vi "Tab Control(Calculator).vi"() -> ()   [LabVIEW 2012]
panel:
  in  "stop":bool
  in  "Tab Control":enum32{"ADD", "SUB", "MUL", "DIV"}(tab)
  out "Result":dbl
  in  "No2":dbl
  in  "NO1":dbl
  in  "NO1 2":dbl
  in  "No2 2":dbl
  out "Result 2":dbl
  in  "NO1 3":dbl
  in  "No2 3":dbl
  out "Result 3":dbl
  in  "NO1 4":dbl
  in  "No2 4":dbl
  out "Result 4":dbl
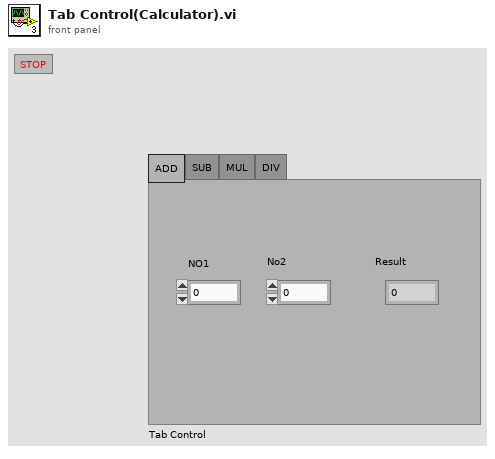
[diagram p1: front panel]
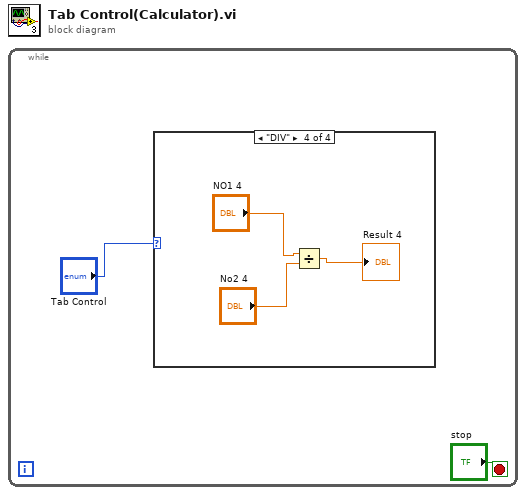
[diagram p0: block diagram]
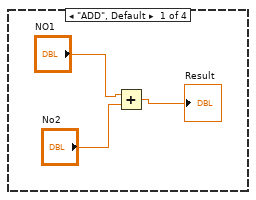
[diagram p2: hidden frame]
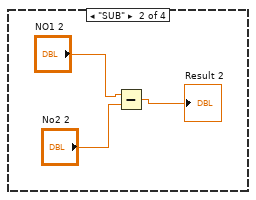
[diagram p3: hidden frame]
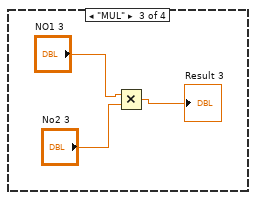
[diagram p4: hidden frame]
diagram:
  n1 = while {
    stop <- "stop" stop-if-true
    n2 = case shown="\"DIV\"" "Tab Control" {
      frame "ADD", Default {
        n3 = Add(x="NO1", y="No2") -> (x+y=→"Result":dbl)
      }
      frame "SUB" {
        n4 = Subtract(x="NO1 2", y="No2 2") -> (x-y=→"Result 2":dbl)
      }
      frame "MUL" {
        n5 = Multiply(x="NO1 3", y="No2 3") -> (x*y=→"Result 3":dbl)
      }
      frame "DIV" {
        n6 = Divide(x="NO1 4", y="No2 4") -> (x/y=→"Result 4":dbl)
      }
    }
  }
